vi "UE9 6-PWM8 Example.vi"(8 "error in":errorcluster, 9 "FIO0 Duty Cycle [%]":dbl=50.0 format="%.1f", 10 "8-bit PWM Frequency [Hz]":dbl=1000.0 format="%.2f") -> (2 "Actual 8-bit Frequency":dbl format="%.1f")   [LabVIEW 2021]
panel:
  in  "FIO5 Duty Cycle [%]":dbl=50.0 format="%.1f"
  in  "FIO4 Duty Cycle [%]":dbl=50.0 format="%.1f"
  in  "FIO3 Duty Cycle [%]":dbl=50.0 format="%.1f"
  out "Update":bool
  out "Timer Value Array":u16[](array[numeric])
  in  "FIO2 Duty Cycle [%]":dbl=50.0 format="%.1f"
  in  "FIO1 Duty Cycle [%]":dbl=50.0 format="%.1f"
  in  "stop":bool
  in  "FirstFound":bool=TRUE
  in  "Address":string="1"
  in  "ConnectionType":u16(ring) items=["LJ_ctUSB", "LJ_ctETHERNET"]
  out "TimerClockDivisor":u8
  out "TimerClockBase":dbl format="%.2f"
  out "Error Message":string
  # "Demonstrates 6 channels of 8-bit PWM output on FIO0-FIO5.\nTimer clock, and timer clock divisor, are chosen to get as close as possible to the desired PWM frequency.\nFor 2.9<=f<=732.4, system clock is used for timer clock.\nFor f<2.9, fixed 750kHz timer clock is used for timer clock."
  # "This VI allows the duty cycles to\nbe changed while the VI is running."
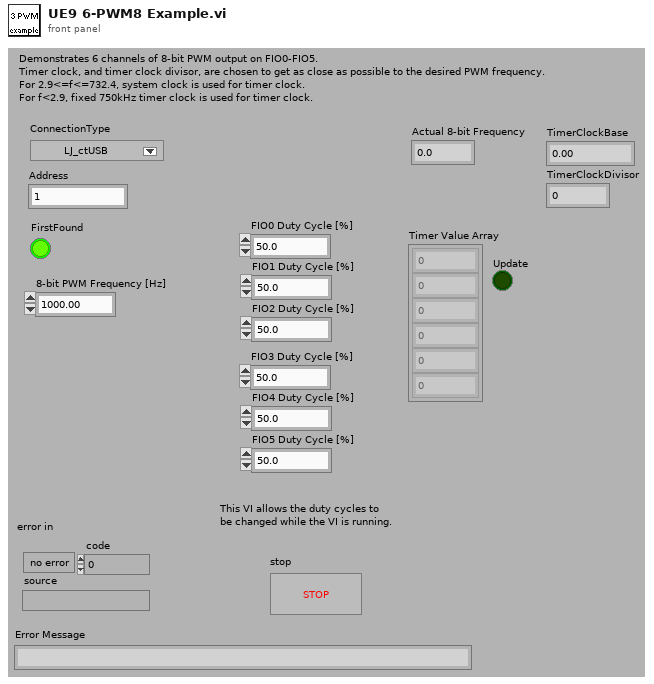
[diagram p1: front panel]
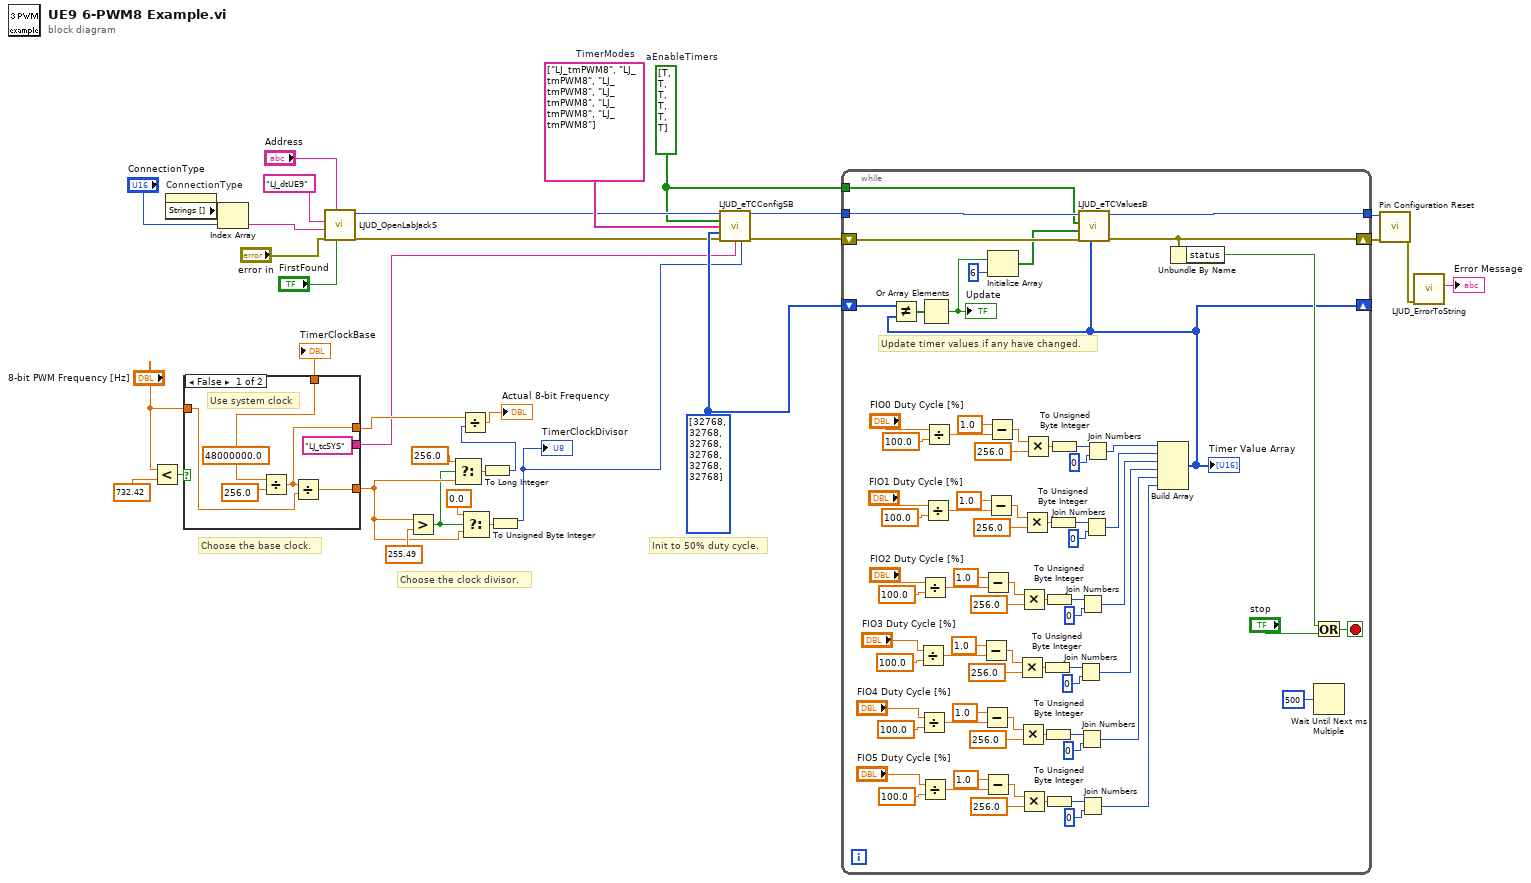
[diagram p0: block diagram]
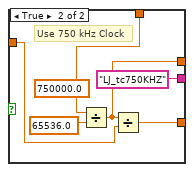
[diagram p2: hidden frame]
diagram:
  w1 = bool[] [TRUE, TRUE, TRUE, TRUE, TRUE, TRUE]  # aEnableTimers
  w6 = string[] ["LJ_tmPWM8", "LJ_tmPWM8", "LJ_tmPWM8", "LJ_tmPWM8", "LJ_tmPWM8", "LJ_tmPWM8"]  # TimerModes
  w10 = u16[] [32768, 32768, 32768, 32768, 32768, 32768] ("TimerValues")
  # "Choose the clock divisor."
  # "Choose the base clock."
  # "Init to 50% duty cycle."
  n1 = Less?(x="8-bit PWM Frequency [Hz]", y=732.42) -> (x < y?=w28:bool)
  n2 = property on="ConnectionType" class="Ring (strict)"() -> ("Strings []"=w15:string[])  [unwired: 2 in, 2 out]
  n3 = case shown="False" w28 {
    tunnel: "8-bit PWM Frequency [Hz]" -> [w39 w45]
    tunnel: [w38 w44] -> w22
    tunnel: [w36 w43] -> w18
    tunnel: [w37 w42] -> w19
    tunnel: ["LJ_tcSYS" ("Timer Clock Base") "LJ_tc750KHZ" ("Timer Clock Base")] -> w3
    frame False {
      w37 = 48000000.0 ("x")
      # "Use system clock"
      n4 = Divide(x=w37, y=256.0) -> (x/y=w36:dbl)
      n5 = Divide(x=w36, y=w39) -> (x/y=w38:dbl)
    }
    frame True {
      w42 = 750000.0 ("x")
      # "Use 750 kHz Clock"
      n6 = Divide(x=w42, y=65536.0) -> (x/y=w43:dbl)
      n7 = Divide(x=w43, y=w45) -> (x/y=w44:dbl)
    }
  }
  "TimerClockBase" <- w19
  n8 = Index Array(array=w15, index="ConnectionType") -> (element=w13:string)
  n9 = call "LJUD_OpenLabJackS.vi"("FirstFound"="FirstFound", "Address"="Address", "error in"="error in", "ConnectionType"=w13, "DeviceType"="LJ_dtUE9") -> ("error out"=w4:errorcluster, "Handle"=w5:i32)  [unwired: 4 in, 1 out]
  n10 = Greater?(x=w22, y=255.49) -> (0:w21:bool)
  n11 = Select(t=256.0, s=w21, f=w22) -> (s? t:f=w24:dbl)
  n12 = Select(t=0.0, s=w21, f=w22) -> (s? t:f=w30:dbl)
  n13 = To Long Integer(number=w24) -> (32bit integer=w20:i32)
  n14 = Divide(x=w18, y=w20) -> (x/y=→"Actual 8-bit Frequency":dbl)
  n15 = To Unsigned Byte Integer(number=w30) -> (unsigned 8bit integer=w2:u8)
  "TimerClockDivisor" <- w2
  n16 = call "LJUD_eTCConfigSB.vi"("Handle In"=w5, "aEnableTimers"=w1, "aTimerModes"=w6, "aTimerValues"=w10, "error in"=w4, "TimerClockBase"=w3, "TimerClockDivisor"=w2) -> ("Handle Out"=w12:i32, "error out"=w11:errorcluster)  [unwired: 7 in]
  n17 = while {
    tunnel: w1 -> [w87]
    tunnel: [w92] -> w9
    shift-left: w10 -> [w95]
    shift-right: [w85] -> _
    tunnel: w12 -> [w98]
    shift-left: w11 -> [w99]
    shift-right: [w96] -> w8
    stop <- w97 stop-if-true
    # "Update timer values if any have changed."
    n18 = Divide(x="FIO3 Duty Cycle [%]", y=100.0) -> (x/y=w73:dbl)
    n19 = Divide(x="FIO4 Duty Cycle [%]", y=100.0) -> (x/y=w68:dbl)
    n20 = Divide(x="FIO2 Duty Cycle [%]", y=100.0) -> (x/y=w119:dbl)
    n21 = Divide(x="FIO5 Duty Cycle [%]", y=100.0) -> (x/y=w57:dbl)
    n22 = Divide(x="FIO1 Duty Cycle [%]", y=100.0) -> (x/y=w110:dbl)
    n23 = Divide(x="FIO0 Duty Cycle [%]", y=100.0) -> (x/y=w105:dbl)
    n24 = Subtract(x=1.0, y=w73) -> (x-y=w75:dbl)
    n25 = Subtract(x=1.0, y=w68) -> (x-y=w66:dbl)
    n26 = Subtract(x=1.0, y=w119) -> (x-y=w117:dbl)
    n27 = Subtract(x=1.0, y=w57) -> (x-y=w59:dbl)
    n28 = Subtract(x=1.0, y=w110) -> (x-y=w112:dbl)
    n29 = Subtract(x=1.0, y=w105) -> (x-y=w103:dbl)
    n30 = Multiply(x=w75, y=256.0) -> (x*y=w78:dbl)
    n31 = Multiply(x=w66, y=256.0) -> (x*y=w63:dbl)
    n32 = Multiply(x=w117, y=256.0) -> (x*y=w114:dbl)
    n33 = Multiply(x=w59, y=256.0) -> (x*y=w62:dbl)
    n34 = Multiply(x=w112, y=256.0) -> (x*y=w48:dbl)
    n35 = Multiply(x=w103, y=256.0) -> (x*y=w47:dbl)
    n36 = To Unsigned Byte Integer(number=w78) -> (unsigned 8bit integer=w76:u8)
    n37 = To Unsigned Byte Integer(number=w63) -> (unsigned 8bit integer=w65:u8)
    n38 = To Unsigned Byte Integer(number=w114) -> (unsigned 8bit integer=w116:u8)
    n39 = To Unsigned Byte Integer(number=w62) -> (unsigned 8bit integer=w60:u8)
    n40 = To Unsigned Byte Integer(number=w48) -> (unsigned 8bit integer=w82:u8)
    n41 = To Unsigned Byte Integer(number=w47) -> (unsigned 8bit integer=w83:u8)
    n42 = Join Numbers(hi=w76, lo=u8 0) -> ((hi.lo)=w51:u16)
    n43 = Join Numbers(hi=w65, lo=u8 0) -> ((hi.lo)=w50:u16)
    n44 = Join Numbers(hi=w116, lo=u8 0) -> ((hi.lo)=w100:u16)
    n45 = Join Numbers(hi=w60, lo=u8 0) -> ((hi.lo)=w49:u16)
    n46 = Join Numbers(hi=w82, lo=u8 0) -> ((hi.lo)=w80:u16)
    n47 = Join Numbers(hi=w83, lo=u8 0) -> ((hi.lo)=w79:u16)
    n48 = Build Array(w79, w80, w100, w51, w50, w49) -> (w85:u16[])
    "Timer Value Array" <- w85
    n49 = Not Equal?(x=w95, y=w85) -> (x != y?=w94:bool[])
    n50 = Or Array Elements(Boolean array=w94) -> (logical OR=w93:bool)
    "Update" <- w93
    n51 = Initialize Array(w93, 6 ("Dimension Size")) -> (w86:bool[])
    n52 = call "LJUD_eTCValuesB.vi"("aTimerValues Write"=w85, "error in"=w99, "aUpdateResetTimers"=w86, "aReadTimers"=w87, "Handle In"=w98) -> ("error out"=w96:errorcluster, "Handle Out"=w92:i32)  [unwired: 3 in, 2 out]
    n53 = Unbundle By Name(w96) -> ("status"=w91:bool)
    n54 = Or(x=w91, y="stop") -> (x .or. y?=w97:bool)
    n55 = Wait Until Next ms Multiple(millisecond multiple=u32 500) -> ()  [unwired: 1 out]
  }
  n56 = call "Pin Configuration Reset.vi"("error in"=w8, "Handle In"=w9) -> ("error out"=w7:errorcluster)  [unwired: 8 in, 1 out]
  n57 = call "LJUD_ErrorToString.vi"("error in"=w7) -> ("String"=→"Error Message":string)  [unwired: 10 in]
